vi "Create Fan Tasks.vi"(4 "Error In":errorcluster, 7 "DAQmx Device Name":tag="Dev2") -> (0 "Error Out":errorcluster, 3 "Hellicopter Tasks Output":T1)   [LabVIEW 2017]
uses:
  <vilib>/DAQmx/read.llb/DAQmx Read (Analog 2D DBL NChan NSamp).vi
  <vilib>/DAQmx/create/channels.llb/DAQmx Create Channel (AI-Voltage-Basic).vi
  <vilib>/DAQmx/configure/timing.llb/DAQmx Timing (Sample Clock).vi
  <vilib>/DAQmx/create/channels.llb/DAQmx Create Channel (CI-Position-Angular Encoder).vi
  <vilib>/DAQmx/miscellaneous.llb/DAQmx Fill In Error Info.vi
  <vilib>/DAQmx/create/channels.llb/DAQmx Create Channel (AO-Voltage-Basic).vi
  <vilib>/DAQmx/create/channels.llb/DAQmx Create Channel (DO-Digital Output).vi
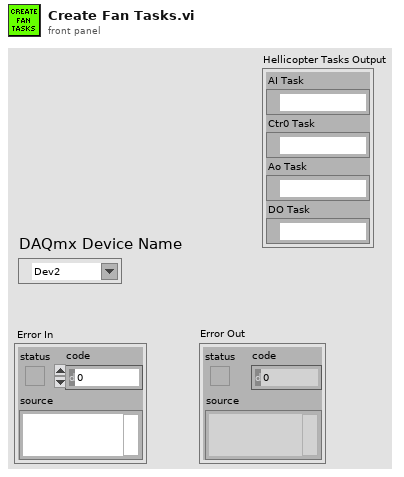
[diagram p1: front panel]
types:
  T1 = cluster{"AI Task":refnum<k21>, "Ctr0 Task":refnum<k21>, "Ao Task":refnum<k21>, "DO Task":refnum<k21>}
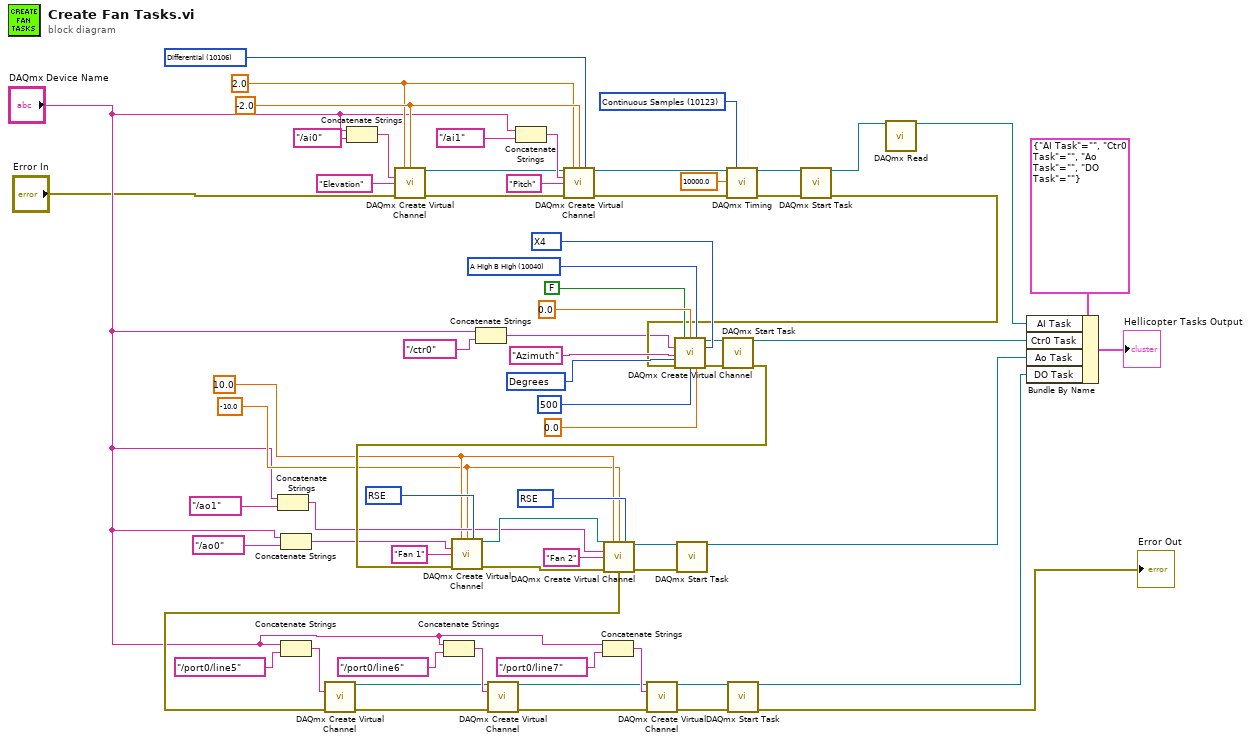
[diagram p0: block diagram]
diagram:
  w7 = -10.0 ("minimum value")
  w8 = 10.0 ("maximum value")
  w68 = 10083 items=["Default"=-1, "RSE"=10083, "Differential"=10106, "Pseudodifferential"=12529] ("output terminal configuration")
  w61 = 10083 items=["Default"=-1, "RSE"=10083, "Differential"=10106, "Pseudodifferential"=12529] ("output terminal configuration")
  w58 = 10146 items=["Degrees"=10146, "Radians"=10273, "Ticks"=10304, "From Custom Scale"=10065] ("units")
  w55 = 10040 items=["A High B High"=10040, "A High B Low"=10041, "A Low B High"=10042, "A Low B Low"=10043] ("z index phase")
  w54 = 10092 items=["X1"=10090, "X2"=10091, "X4"=10092, "Two Pulse Counting"=10313] ("decoding type")
  w49 = 10123 items=["Finite Samples"=10178, "Continuous Samples"=10123, "Hardware Timed Single Point"=12522] ("sample mode")
  w45 = 10106 items=["default"=-1, "RSE"=10083, "NRSE"=10078, "Differential"=10106, "Pseudodifferential"=12529] ("input terminal configuration")
  w6 = -2.0 ("minimum value")
  w5 = 2.0 ("maximum value")
  n1 = Concatenate Strings("DAQmx Device Name", tag "/ao1" ("physical channels")) -> (w32:string)
  n2 = Concatenate Strings("DAQmx Device Name", tag "/ao0" ("physical channels")) -> (w33:string)
  n3 = Concatenate Strings("DAQmx Device Name", tag "/port0/line5" ("lines")) -> (w28:string)
  n4 = Concatenate Strings("DAQmx Device Name", tag "/ai0" ("physical channels")) -> (w14:string)
  n5 = call-poly <vilib>:"DAQmx Create Virtual Channel.vi"("maximum value"=w5, "minimum value"=w6, "physical channels"=w14, "name to assign"="Elevation", "error in"="Error In") -> ("task out"=w11:refnum<k21>, "error out"=w10:errorcluster)  [unwired: 9 in]
  n6 = Concatenate Strings("DAQmx Device Name", tag "/port0/line6" ("lines")) -> (w27:string)
  n7 = Concatenate Strings("DAQmx Device Name", tag "/ctr0" ("counter")) -> (w36:string)
  n8 = Concatenate Strings("DAQmx Device Name", tag "/ai1" ("physical channels")) -> (w30:string)
  n9 = call-poly <vilib>:"DAQmx Create Virtual Channel.vi"("task in"=w11, "maximum value"=w5, "minimum value"=w6, "input terminal configuration"=w45, "physical channels"=w30, "name to assign"="Pitch", "error in"=w10) -> ("task out"=w46:refnum<k21>, "error out"=w47:errorcluster)  [unwired: 7 in]
  n10 = Concatenate Strings("DAQmx Device Name", tag "/port0/line7" ("lines")) -> (w26:string)
  n11 = call-poly <vilib>:"DAQmx Timing.vi"("task/channels in"=w46, "sample mode"=w49, "rate"=10000.0, "error in"=w47) -> ("task out"=w3:refnum<k21>, "error out"=w52:errorcluster)  [unwired: 10 in]
  n12 = call <vilib>:"DAQmx Start Task.vi"("task/channels in"=w3, "error in"=w52) -> ("task out"=w40:refnum<k21>, "error out"=w43:errorcluster)  [unwired: 12 in]
  n13 = call-poly <vilib>:"DAQmx Create Virtual Channel.vi"("z index enable"=FALSE, "z index value"=0.0, "z index phase"=w55, "counter"=w36, "decoding type"=w54, "name to assign"="Azimuth", "units"=w58, "error in"=w43, "pulses per revolution"=u32 500, "initial angle"=0.0) -> ("task out"=w53:refnum<k21>, "error out"=w57:errorcluster)  [unwired: 4 in]
  n14 = call <vilib>:"DAQmx Start Task.vi"("task/channels in"=w53, "error in"=w57) -> ("task out"=w39:refnum<k21>, "error out"=w42:errorcluster)  [unwired: 12 in]
  n15 = call-poly <vilib>:"DAQmx Create Virtual Channel.vi"("maximum value"=w8, "minimum value"=w7, "output terminal configuration"=w68, "physical channels"=w33, "name to assign"="Fan 1", "error in"=w42) -> ("task out"=w66:refnum<k21>, "error out"=w67:errorcluster)  [unwired: 8 in]
  n16 = call-poly <vilib>:"DAQmx Create Virtual Channel.vi"("task in"=w66, "maximum value"=w8, "minimum value"=w7, "output terminal configuration"=w61, "physical channels"=w32, "name to assign"="Fan 2", "error in"=w67) -> ("task out"=w63:refnum<k21>, "error out"=w64:errorcluster)  [unwired: 7 in]
  n17 = call <vilib>:"DAQmx Start Task.vi"("task/channels in"=w63, "error in"=w64) -> ("task out"=w38:refnum<k21>, "error out"=w19:errorcluster)  [unwired: 12 in]
  n18 = call-poly <vilib>:"DAQmx Create Virtual Channel.vi"("lines"=w28, "error in"=w19) -> ("task out"=w23:refnum<k21>, "error out"=w20:errorcluster)  [unwired: 12 in]
  n19 = call-poly <vilib>:"DAQmx Create Virtual Channel.vi"("task in"=w23, "lines"=w27, "error in"=w20) -> ("task out"=w22:refnum<k21>, "error out"=w21:errorcluster)  [unwired: 11 in]
  n20 = call-poly <vilib>:"DAQmx Create Virtual Channel.vi"("task in"=w22, "lines"=w26, "error in"=w21) -> ("task out"=w16:refnum<k21>, "error out"=w18:errorcluster)  [unwired: 11 in]
  n21 = call <vilib>:"DAQmx Start Task.vi"("task/channels in"=w16, "error in"=w18) -> ("task out"=w15:refnum<k21>, "error out"=→"Error Out":errorcluster)  [unwired: 12 in]
  n22 = call-poly <vilib>:"DAQmx Read.vi"("task/channels in"=w40) -> ("task out"=w1:refnum<k21>)  [unwired: 12 in, 2 out]
  n23 = Bundle By Name(cluster=T1 {"AI Task"="", "Ctr0 Task"="", "Ao Task"="", "DO Task"=""}, "AI Task"=w1, "Ctr0 Task"=w39, "Ao Task"=w38, "DO Task"=w15) -> (→"Hellicopter Tasks Output":T1)
